vi "Read_DaQ_channels.vi"() -> ()   [LabVIEW 2015]
doc: "Use this template to build a producer/consumer design pattern with events to produce queue items. Use this design pattern instead of the User Interface Event Handler pattern for user interfaces when you want to execute code asynchronously in response to an event without slowing the user interface responsiveness."
uses:
  <vilib>/DAQmx/read.llb/DAQmx Read.vi
  <vilib>/DAQmx/read.llb/DAQmx Read (Analog 1D DBL NChan 1Samp).vi
  <vilib>/DAQmx/create/channels.llb/DAQmx Create Channel (AI-Voltage-Basic).vi
  <vilib>/DAQmx/configure/timing.llb/DAQmx Timing (Sample Clock).vi
  <vilib>/DAQmx/miscellaneous.llb/DAQmx Fill In Error Info.vi
panel:
  in  "minimum value":dbl=-5.0 format="%0.2f"
  in  "maximum value":dbl=5.0 format="%0.2f"
  out "Difference":dbl[](graph)
  out "U+, U-":dbl[][](graph)
  out "element 3":dbl
  out "element 2":dbl
  out "element":dbl
  in  "stop 2":bool
  in  "Enqueue Element":bool
  in  "stop":bool
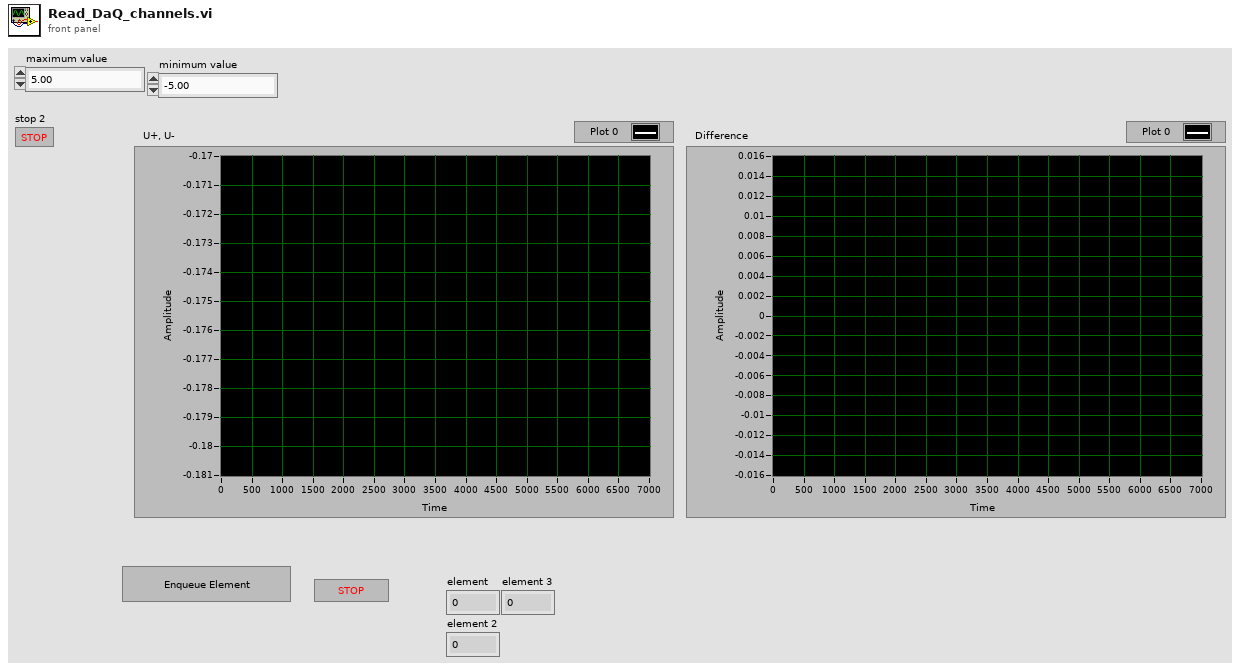
[diagram p1: front panel]
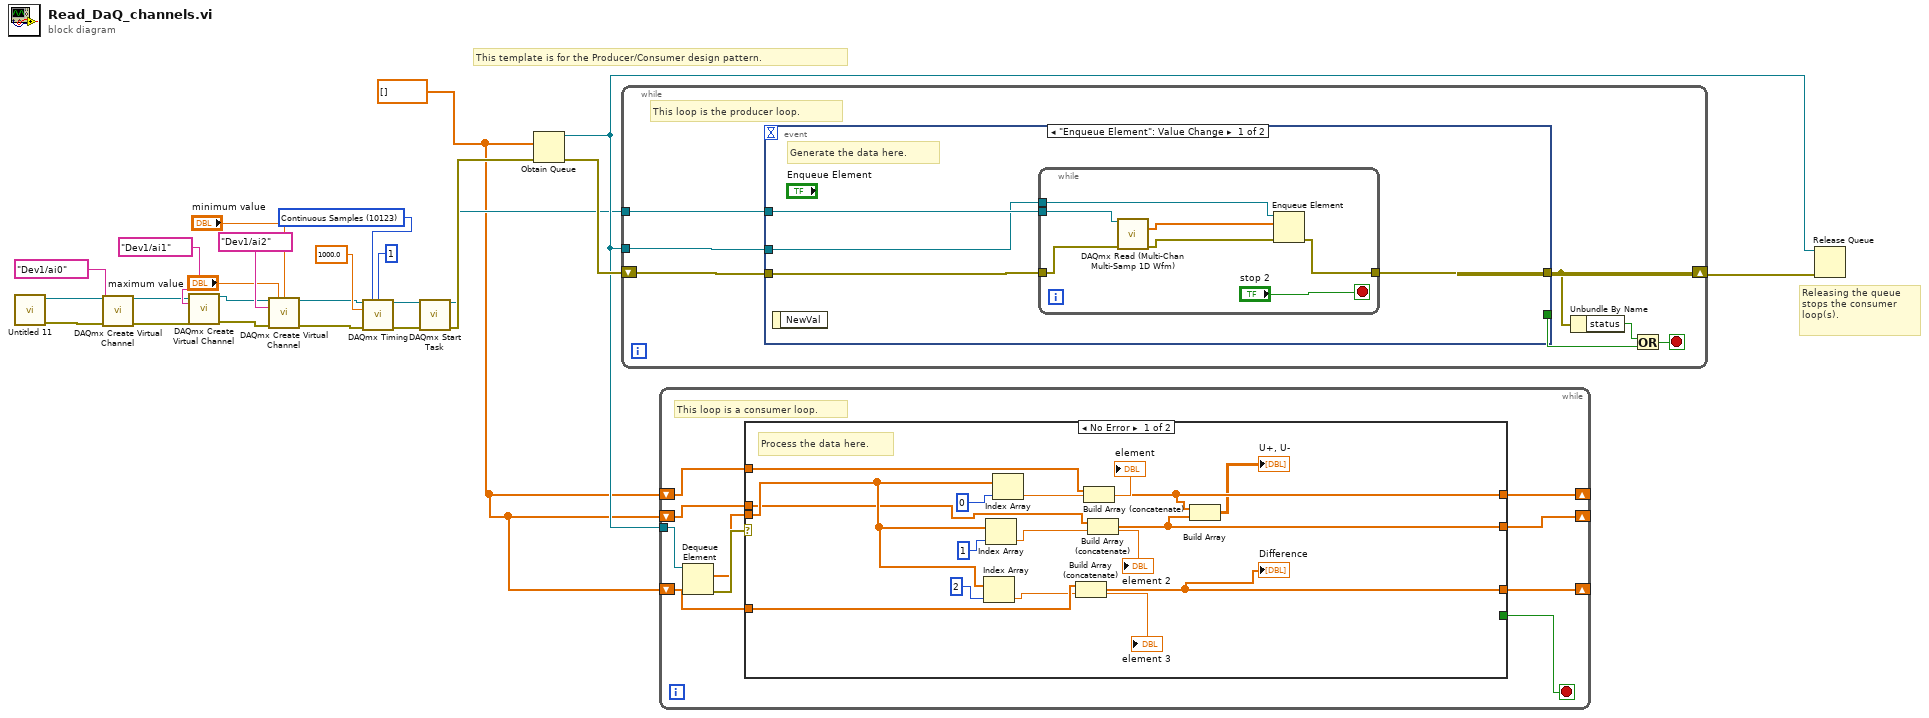
[diagram p0: block diagram]
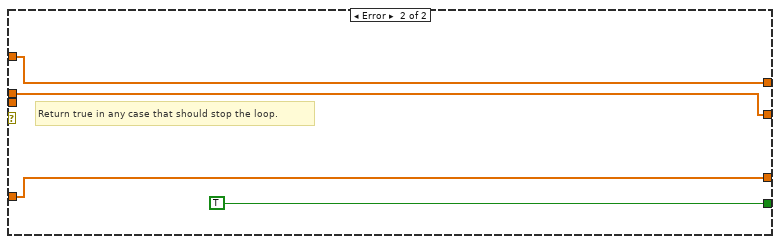
[diagram p2: hidden frame]
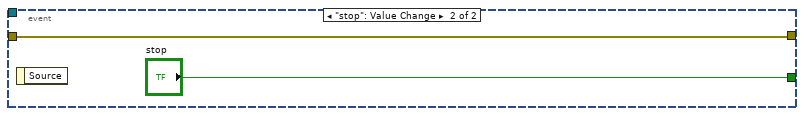
[diagram p3: hidden frame]
diagram:
  w3 = dbl[] [] ("data")
  w6 = 10123 items=["Finite Samples"=10178, "Continuous Samples"=10123, "Hardware Timed Single Point"=12522] ("sample mode")
  # "Releasing the queue stops the consumer loop(s)."
  # "This template is for the Producer/Consumer design pattern."
  n1 = call "Untitled 11.vi"() -> ("error out"=w10:errorcluster, "task out"=w7:refnum<k21>)  [unwired: 10 in]
  n2 = call-poly <vilib>:"DAQmx Create Virtual Channel.vi"("task in"=w7, "physical channels"=tag "Dev1/ai0", "error in"=w10) -> ("task out"=w8:refnum<k21>, "error out"=w11:errorcluster)  [unwired: 11 in]
  n3 = call-poly <vilib>:"DAQmx Create Virtual Channel.vi"("task in"=w8, "physical channels"=tag "Dev1/ai1", "error in"=w11) -> ("task out"=w9:refnum<k21>, "error out"=w12:errorcluster)  [unwired: 11 in]
  n4 = call-poly <vilib>:"DAQmx Create Virtual Channel.vi"("task in"=w9, "maximum value"="maximum value", "minimum value"="minimum value", "physical channels"=tag "Dev1/ai2", "error in"=w12) -> ("task out"=w16:refnum<k21>, "error out"=w18:errorcluster)  [unwired: 9 in]
  n5 = call-poly <vilib>:"DAQmx Timing.vi"("task/channels in"=w16, "sample mode"=w6, "samples per channel"=1, "rate"=1000.0, "error in"=w18) -> ("task out"=w17:refnum<k21>, "error out"=w19:errorcluster)  [unwired: 9 in]
  n6 = call <vilib>:"DAQmx Start Task.vi"("task/channels in"=w17, "error in"=w19) -> ("task out"=w4:refnum<k21>, "error out"=w5:errorcluster)  [unwired: 12 in]
  n7 = Obtain Queue(element data type=w3, error in (no error)=w5) -> (queue out=w22:refnum<queue>, error out=w24:errorcluster)  [unwired: 3 in, 1 out]
  n8 = while {
    shift-right: [w27] -> w23
    shift-left: w24 -> [w30]
    tunnel: w22 -> [w31]
    tunnel: w4 -> [w25]
    stop <- w28 stop-if-true
    # "This loop is the producer loop."
    n9 = event shown="[0] \"Enqueue Element\": Value Change" {
      selector: _ -> [_ _]
      dyn-events: _ -> [_ _]
      timeout: _ -> [_ _]
      tunnel: w31 -> [w34 _]
      tunnel: w30 -> [w33 w43]
      tunnel: [w32 w43] -> w27
      tunnel: [_ "stop"] -> w29
      tunnel: w25 -> [w35 _]
      event "Enqueue Element": Value Change {
        # "Generate the data here."
        n10 = event-data() -> ()  [unwired: 1 in, 1 out]
        n11 = while {
          tunnel: w33 -> [w40]
          tunnel: w35 -> [w41]
          tunnel: w34 -> [w38]
          tunnel: [w36] -> w32
          stop <- "stop 2" stop-if-true
          n12 = call-poly "DAQmx Read (Multi-Chan Multi-Samp 1D Wfm).vi"("task/channels in"=w41, "error in"=w40) -> ("data"=w39:dbl[], "error out"=w37:errorcluster)  [unwired: 11 in, 1 out]
          n13 = Enqueue Element(queue=w38, element=w39, error in (no error)=w37) -> (error out=w36:errorcluster)  [unwired: 1 in, 2 out]
        }
      }
      event "stop": Value Change {
        n14 = event-data() -> ()  [unwired: 1 in, 1 out]
      }
    }
    n15 = Unbundle By Name(w27) -> ("status"=w26:bool)
    n16 = Or(x=w26, y=w29) -> (x .or. y?=w28:bool)
  }
  n17 = while {
    tunnel: w22 -> [w54]
    shift-right: [w50] -> _
    shift-left: w3 -> [w49]
    shift-right: [w48] -> _
    shift-left: w3 -> [w47]
    shift-right: [w46] -> _
    shift-left: w3 -> [w45]
    stop <- w51 stop-if-true
    # "This loop is a consumer loop."
    n18 = Dequeue Element(queue=w54) -> (element=w52:dbl[], error out=w53:errorcluster)  [unwired: 2 in, 2 out]
    n19 = case shown="No Error" w53 {
      tunnel: w52 -> [w65 _]
      tunnel: [_ TRUE] -> w51
      tunnel: [w58 w71] -> w50
      tunnel: w49 -> [w62 w71]
      tunnel: [w57 w69] -> w48
      tunnel: w47 -> [w61 w69]
      tunnel: [w55 w70] -> w46
      tunnel: w45 -> [w60 w70]
      frame No Error {
        # "Process the data here."
        n20 = Index Array(array=w65, index=2) -> (element=w59:dbl)
        "element 3" <- w59
        n21 = Index Array(array=w65, index=1 ("length")) -> (element=w63:dbl)
        "element 2" <- w63
        n22 = Index Array(array=w65, index=0) -> (element=w64:dbl)
        "element" <- w64
        n23 = Build Array (concatenate)(w60, w59) -> (w55:dbl[])
        "Difference" <- w55
        n24 = Build Array (concatenate)(w62, w64) -> (w58:dbl[])
        n25 = Build Array (concatenate)(w61, w63) -> (w57:dbl[])
        n26 = Build Array(w58, w57) -> (→"U+, U-":dbl[][])
      }
      frame Error {
        # "Return true in any case that should stop the loop."
      }
    }
  }
  n27 = Release Queue(queue=w22, error in (no error)=w23) -> ()  [unwired: 1 in, 3 out]
